vi "Read Labels.vi"(8 "error in (no error)":errorcluster, 11 "Sample in":refnum<class "Sample.lvclass">) -> (0 "error out":errorcluster, 2 "Labels":map{string, string}(c390), 3 "Sample out":refnum<class "Sample.lvclass">)   [LabVIEW 2020, in "Metrics.lvlib" / "Sample.lvclass"]
uses:
  Sample.lvclass
  Sample.lvclass/Sample.ctl
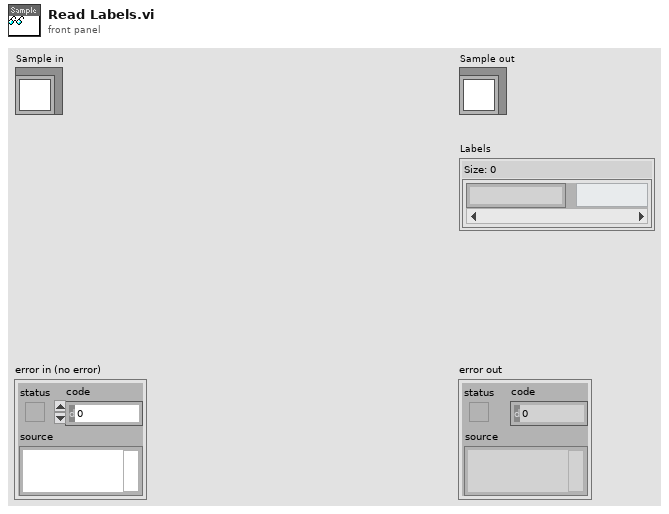
[diagram p1: front panel]
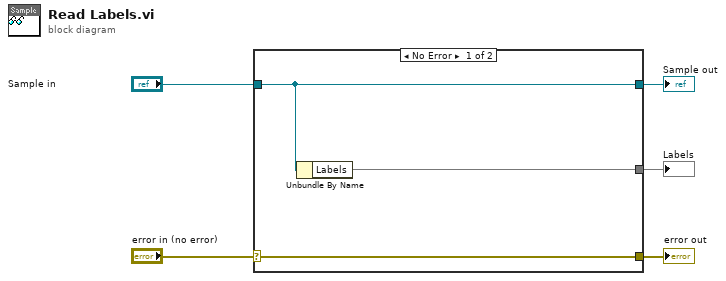
[diagram p0: block diagram]
diagram:
  n1 = case shown="No Error" "error in (no error)" {
    selector: "error in (no error)" -> [w8 w9]
    tunnel: [w8 w9] -> w4
    tunnel: [w7 w10] -> w2
    tunnel: "Sample in" -> [w7 w10]
    tunnel: [w6 _] -> w1
    frame No Error {
      n2 = Unbundle By Name(w7) -> ("Labels"=w6:map{string, string})
    }
    frame Error {
    }
  }
  "error out" <- w4
  "Sample out" <- w2
  "Labels" <- w1
